vi "3-10.vi"   [LabVIEW 2022 SP3]
types:
  T1 = enum16{"open", "replace", "create", "open or create", "replace or create", "replace or create with confirmation"}
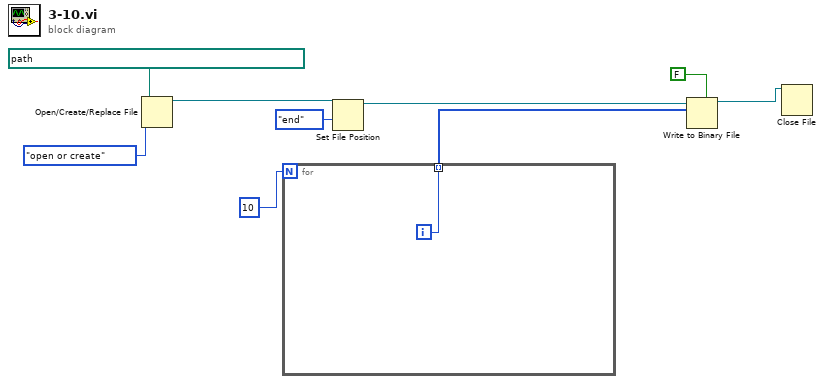
[diagram p0: block diagram]
diagram:
  n1 = Open/Create/Replace File(file path (use dialog)=path "C:/Users/Administrator/Desktop/实验三/test2.bin" ("文件路径（使用对话框）"), operation (0:open)=T1."open or create" ("操作(0:open)")) -> (refnum out=w6:refnum<file>)  [unwired: 4 in, 2 out]
  n2 = for {
    N: 10 -> [_]
    tunnel: [w10] -> w4 mode=indexing
    i -> [w10]
  }
  n3 = Set File Position(refnum=w6, from (0:start)=enum16{"start", "end", "current"}."end" ("自（0:起始）")) -> (refnum out=w3:refnum<file>)  [unwired: 2 in, 1 out]
  n4 = Write to Binary File(file (use dialog)=w3, data=w4, 5:FALSE ("预置数组或字符串大小？ (T)")) -> (refnum out=w1:refnum<file>)  [unwired: 3 in, 2 out]
  n5 = Close File(refnum=w1) -> ()  [unwired: 1 in, 2 out]
